vi "Assign Pixel to Wing Sector (FPGA)V2.vi"(4 "End of Data?":bool, 5 "Valid Data?":bool, 6 "Pixel Intensity In":u8, 7 "Right Wing?":bool, 8 "Sector Parameters":T1, 9 "Pixel Y":u16, 10 "Pixel X":u16) -> (1 "Pixel Intensity Out":u8, 2 "sector #":u8, 3 "output valid":bool)   [LabVIEW 2013]
uses:
  Sector Parameter Cluster.ctl
  <vilib>/rvi/FXPMathLib/FxpRectToPolar/subVIs/nifxpmath_RectToPolar_SimConfig.ctl
  <vilib>/rvi/FXPMathLib/FxpDiv/subVIs/nifxpmath_Div_SimConfig.ctl
  <vilib>/rvi/FXPMathLib/FxpRectToPolar/simVIs/DllFxpRectToPolarTemp_sub.vi
  <vilib>/rvi/FXPMathLib/FxpDiv/simVIs/DllFxpDivTemp_sub.vi
  <vilib>/rvi/FXPMathLib/FxpSub/XNode/nifxpmath_Sub.xnode
  <vilib>/rvi/FXPMathLib/FxpRectToPolar/XNode/nifxpmath_RectToPolar.xnode
  <vilib>/rvi/FXPMathLib/FxpAdd/XNode/nifxpmath_Add.xnode
  <vilib>/rvi/FXPMathLib/FxpDiv/XNode/nifxpmath_Div.xnode
  <vilib>/rvi/FXPMathLib/sim/FxpSim.dll
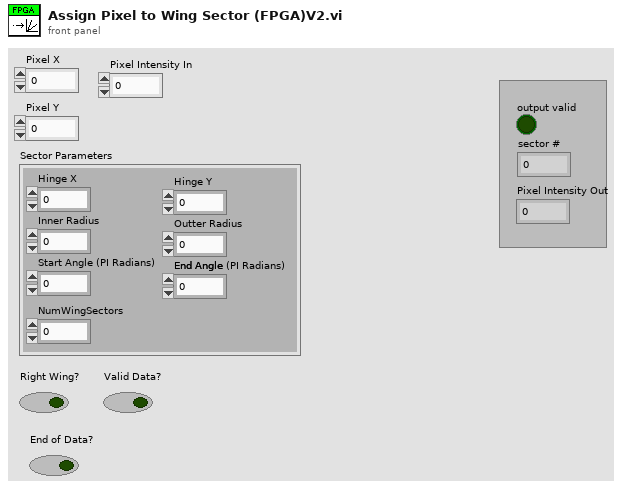
[diagram p1: front panel]
types:
  T1 = typedef "Sector Parameter Cluster.ctl" = cluster{"Start Angle":fxp<+/-,17,2>, "End Angle":fxp<+,17,3>, "Inner Radius":u16, "Outter Radius":u16, "Hinge X":u16, "Hinge Y":u16, "NumWingSectors":u8}
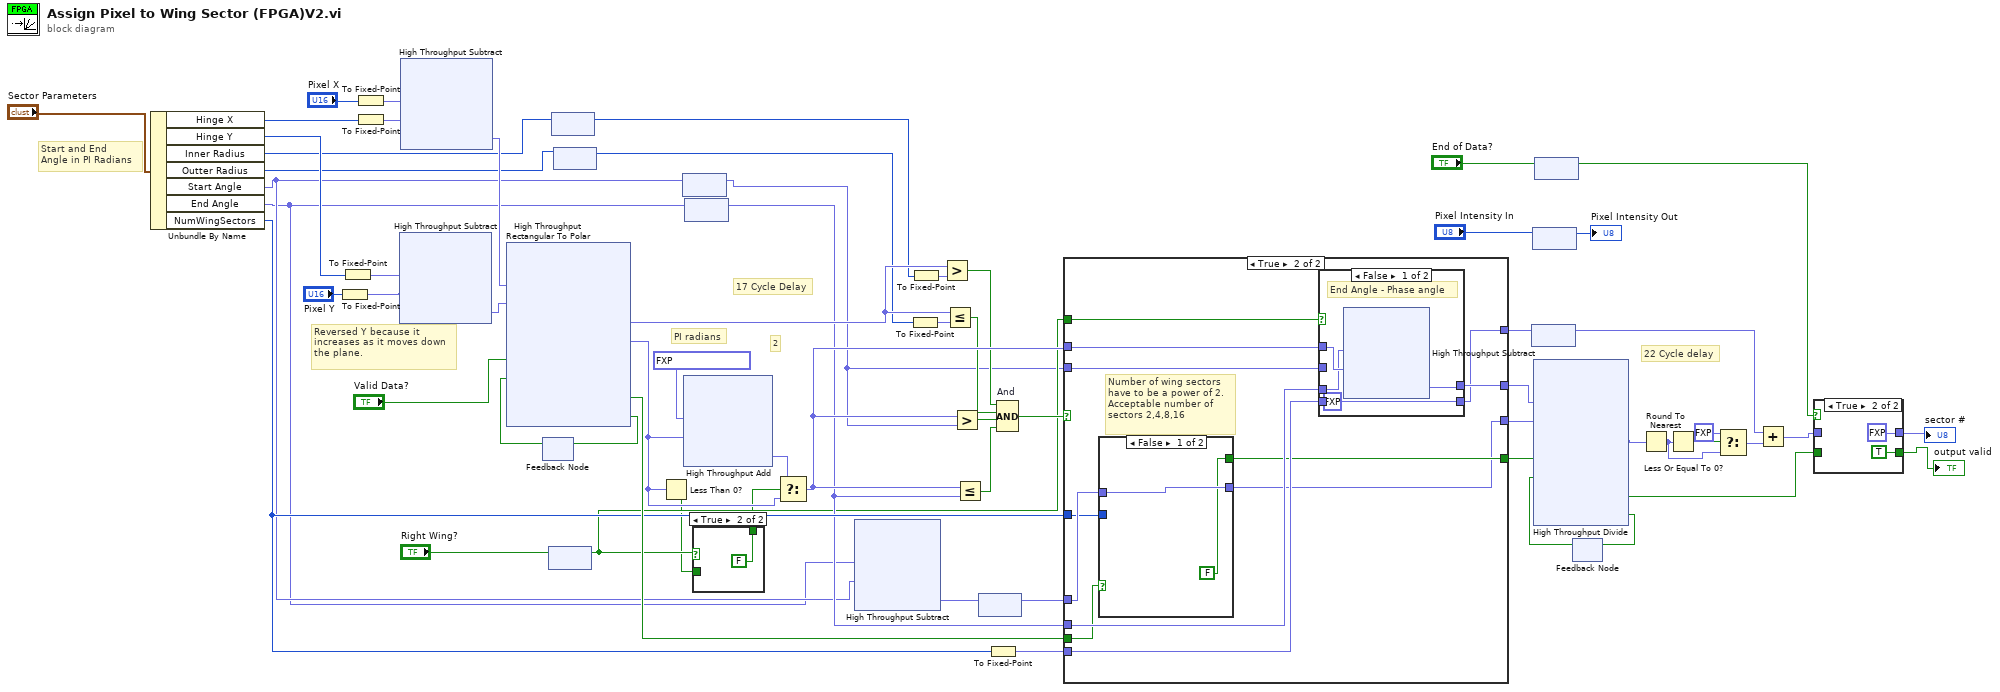
[diagram p0: block diagram]
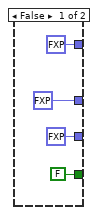
[diagram p4: hidden frame]
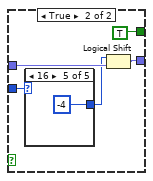
[diagram p5: hidden frame]
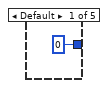
[diagram p6: hidden frame]
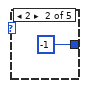
[diagram p7: hidden frame]
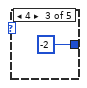
[diagram p8: hidden frame]
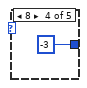
[diagram p9: hidden frame]
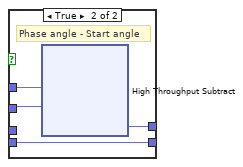
[diagram p10: hidden frame]
diagram:
  # "17 Cycle Delay"
  # "Reversed Y because it\nincreases as it moves down\nthe plane."
  # "PI radians"
  # "22 Cycle delay"
  # "Start and End\nAngle in PI Radians"
  # "2"
  n1 = Unbundle By Name("Sector Parameters") -> ("Hinge X"=w30:u16, "Hinge Y"=w49:u16, "Inner Radius"=w28:u16, "Outter Radius"=w26:u16, "Start Angle"=w12:fxp<+/-,17,2>, "End Angle"=w10:fxp<+,17,3>, "NumWingSectors"=w35:u8)
  n2 = To Fixed-Point(number="Pixel Y") -> (fixed-point=w39:fxp<+,11,11>)  [unwired: 1 in]
  n3 = To Fixed-Point(number=w49) -> (fixed-point=w40:fxp<+,11,11>)  [unwired: 1 in]
  n4 = To Fixed-Point(number="Pixel X") -> (fixed-point=w38:fxp<+,11,11>)  [unwired: 1 in]
  n5 = To Fixed-Point(number=w30) -> (fixed-point=w37:fxp<+,11,11>)  [unwired: 1 in]
  n6 = xnode "High Throughput Subtract"("x"=w40, "y"=w39) -> ("x-y"=w48:fxp<+/-,12,12>)
  n7 = xnode "High Throughput Subtract"("x"=w38, "y"=w37) -> ("x-y"=w47:fxp<+/-,12,12>)
  n8 = feedback #1() -> (w54:bool)  [unwired: 1 in]
  n9 = xnode "High Throughput Rectangular To Polar"("x"=w47, "y"=w48, "input valid"="Valid Data?", "ready for output (T)"=w54) -> ("magnitude"=w62:fxp<+,12,12>, "phase (pi)"=w59:fxp<+/-,16,2>, "output valid"=w36:bool, "ready for input"=w55:bool)
  n10 = feedback-in #1(w55) -> ()
  n11 = feedback #2() -> (w22:bool)  [unwired: 1 in]
  n12 = feedback-in #2("Right Wing?") -> ()
  n13 = feedback #3() -> (w27:u16)  [unwired: 1 in]
  n14 = feedback-in #3(w28) -> ()
  n15 = feedback #4() -> (w25:u16)  [unwired: 1 in]
  n16 = feedback-in #4(w26) -> ()
  n17 = Less Than 0?(x=w59) -> (x < 0?=w20:bool)
  n18 = feedback #5() -> (w11:fxp<+/-,17,2>)  [unwired: 1 in]
  n19 = feedback-in #5(w12) -> ()
  n20 = xnode ("High Throughput Add")("x"=fxp<+/-,16,2> 1.99993896484375 ("y"), "y"=w59) -> ("x+y"=w58:fxp<+/-,17,3>)
  n21 = feedback #6() -> (w24:fxp<+,17,3>)  [unwired: 1 in]
  n22 = feedback-in #6(w10) -> ()
  n23 = case shown="True" w22 {
    tunnel: [w64 FALSE ("s")] -> w21
    tunnel: w20 -> [w64 _]
    frame False {
    }
    frame True {
    }
  }
  n24 = Select(t=w58, s=w21, f=w59) -> (s? t:f=w56:fxp<+/-,17,3>)
  n25 = xnode ("High Throughput Subtract")("x"=w10, "y"=w12) -> ("x-y"=w9:fxp<+/-,17,6>)
  n26 = To Fixed-Point(number=w25) -> (fixed-point=w61:fxp<+,16,16>)  [unwired: 1 in]
  n27 = To Fixed-Point(number=w27) -> (fixed-point=w63:fxp<+,16,16>)  [unwired: 1 in]
  n28 = Greater?(x=w62, y=w63) -> (0:w53:bool)
  n29 = Less Or Equal?(x=w62, y=w61) -> (x <= y?=w52:bool)
  n30 = Greater?(x=w56, y=w11) -> (0:w51:bool)
  n31 = Less Or Equal?(x=w56, y=w24) -> (x <= y?=w50:bool)
  n32 = feedback #7() -> (w8:fxp<+/-,17,6>)  [unwired: 1 in]
  n33 = feedback-in #7(w9) -> ()
  n34 = To Fixed-Point(number=w35) -> (fixed-point=w18:fxp<+,8,8>)  [unwired: 1 in]
  n35 = Compound Arithmetic op=AND "And"(w53, w52, w51, w50) -> (w60:bool)
  n36 = case shown="True" w60 {
    tunnel: w56 -> [_ w81]
    tunnel: w11 -> [_ w80]
    tunnel: [fxp<+/-,17,6> 0.0 ("x-y") w71] -> w44
    tunnel: w24 -> [_ w78]
    tunnel: w18 -> [_ w79]
    tunnel: [fxp<+/-,20,5> 0.0 ("x-y") w77] -> w45
    tunnel: [FALSE ("output valid") w72] -> w43
    tunnel: [fxp<+,8,8> 0.0 w76] -> w41
    tunnel: w8 -> [_ w75]
    tunnel: w36 -> [_ w74]
    tunnel: w35 -> [_ w73]
    tunnel: w22 -> [_ w70]
    frame False {
    }
    frame True {
      # "Number of wing sectors\nhave to be a power of 2.\nAcceptable number of\nsectors 2,4,8,16"
      n37 = case shown="False" w74 {
        tunnel: w73 -> [_ w88]
        tunnel: w75 -> [w83 w87]
        tunnel: [w83 w85] -> w71
        tunnel: [FALSE ("output valid") TRUE ("output valid")] -> w72
        frame False {
        }
        frame True {
          n38 = case shown="16" w88 {
            tunnel: [i16 0 ("y") i16 -1 ("y") i16 -2 ("y") i16 -3 ("y") i16 -4 ("y")] -> w86
            frame Default {
            }
            frame 2 {
            }
            frame 4 {
            }
            frame 8 {
            }
            frame 16 {
            }
          }
          n39 = Logical Shift(y=w86, x=w87) -> (x << y=w85:fxp<+/-,17,6>)
        }
      }
      n40 = case shown="False" w70 {
        tunnel: w81 -> [w96 w101]
        tunnel: w80 -> [_ w100]
        tunnel: [w97 w99] -> w77
        tunnel: w79 -> [_ w98]
        tunnel: [fxp<+,8,8> 0.0 w98] -> w76
        tunnel: w78 -> [w95 _]
        frame False {
          # "End Angle - Phase angle"
          n41 = xnode "High Throughput Subtract"("x"=w95, "y"=w96) -> ("x-y"=w97:fxp<+/-,19,5>)
        }
        frame True {
          # "Phase angle - Start angle"
          n42 = xnode ("High Throughput Subtract")("x"=w101, "y"=w100) -> ("x-y"=w99:fxp<+/-,19,4>)
        }
      }
    }
  }
  n43 = feedback #8() -> (w13:fxp<+,8,8>)  [unwired: 1 in]
  n44 = feedback-in #8(w41) -> ()
  n45 = feedback #9() -> (→"Pixel Intensity Out":u8)  [unwired: 1 in]
  n46 = feedback-in #9("Pixel Intensity In") -> ()
  n47 = feedback #10() -> (w5:bool)  [unwired: 1 in]
  n48 = feedback-in #10("End of Data?") -> ()
  n49 = feedback #11() -> (w42:bool)  [unwired: 1 in]
  n50 = xnode "High Throughput Divide"("x"=w45, "y"=w44, "input valid"=w43, "ready for output (T)"=w42) -> ("x/y"=w15:fxp<+/-,20,16>, "output valid"=w1:bool, "ready for input"=w46:bool)
  n51 = feedback-in #11(w46) -> ()
  n52 = Round To Nearest(number=w15) -> (nearest integer value=w14:fxp<+/-,17,17>)
  n53 = Less Or Equal To 0?(x=w14) -> (x <= 0?=w17:bool)
  n54 = Select(t=fxp<+/-,17,17> 1.0, s=w17, f=w14) -> (s? t:f=w23:fxp<+/-,17,17>)
  n55 = Add(x=w13, y=w23) -> (x+y=w3:fxp<+/-,17,17>)
  n56 = case shown="True" w5 {
    tunnel: [w103 fxp<+/-,17,17> 0.0] -> w4
    tunnel: w3 -> [w103 _]
    tunnel: [w102 TRUE ("output valid")] -> w2
    tunnel: w1 -> [w102 _]
    frame False {
    }
    frame True {
    }
  }
  "output valid" <- w2
  "sector #" <- w4
